vi "Configure Mask Test.vi"(0 "VISA resource name":refnum<visa-resource-name>, 1 "Enable Mask Test (Enable)":bool, 5 "Source (1: Channel 1)":i32(ring) items=["Channel 1", "Channel 2", "Channel 3", "Channel 4", "Function 1", "Function 2", "Function 3", "Function 4"], 7 "Trigger Source (1: Channel 1)":i32(ring) items=["Channel 1", "Channel 2", "Channel 3", "Channel 4"], 9 "Impedance (0: None)":i32(ring) items=["None", "IMP75", "IMP100", "IMP110", "IMP120"], 11 "error in (no error)":errorcluster, 12 "Run":T2 {"Time (1.0 min)" format="%#.1g"; "Run Mode (0: Forever)" items=["Forever", "Waveform", "Time"]}, 13 "Test Options":T3, 14 "Pulse Amplitude":T1) -> (4 "VISA resource name out":refnum<visa-resource-name>, 15 "error out":errorcluster)   [LabVIEW 2009, in "Agilent 8000 Series.lvlib"]
doc: "Configures the Mask test and the parameters required for a mask test. This VI has to be called before calling any other Mask related VIs."
uses:
  Agilent 8000 Series.lvlib
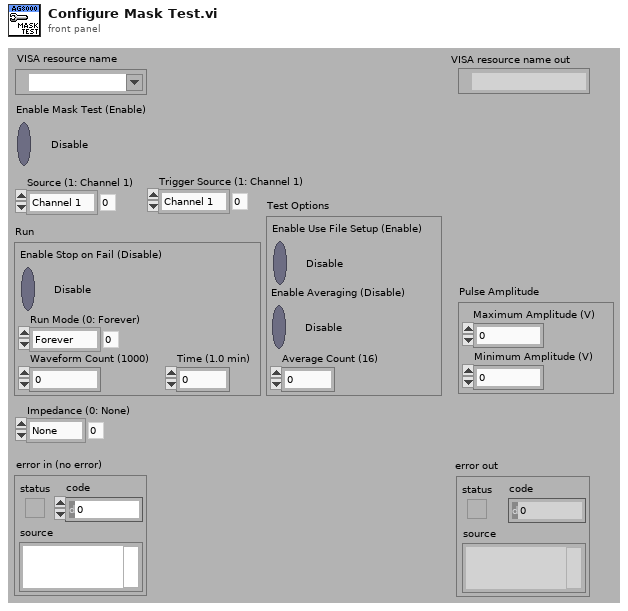
[diagram p1: front panel]
types:
  T1 = cluster{"Maximum Amplitude (V)":dbl, "Minimum Amplitude (V)":dbl}
  T2 = cluster{"Enable Stop on Fail (Disable)":bool, "Run Mode (0: Forever)":i32, "Waveform Count (1000)":u32, "Time (1.0 min)":dbl}
  T3 = cluster{"Enable Averaging (Disable)":bool, "Average Count (16)":u32, "Enable Use File Setup (Enable)":bool}
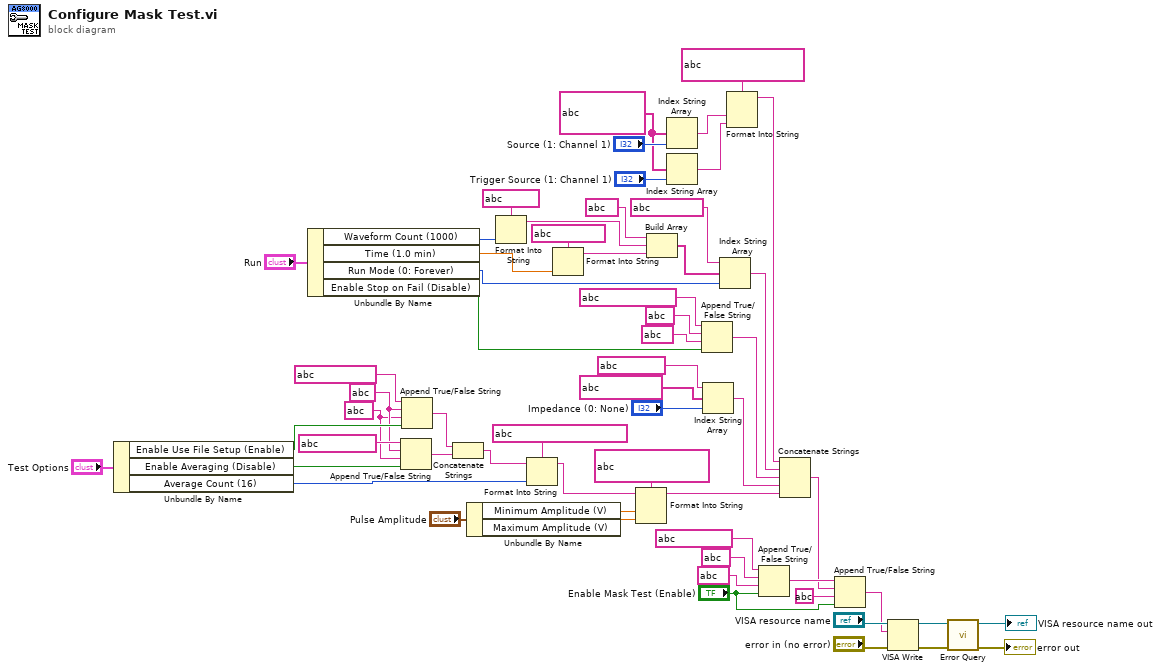
[diagram p0: block diagram]
diagram:
  w1 = string ? ("false string")
  w2 = string ? ("true string")
  w48 = string[] ?
  n1 = Unbundle By Name("Test Options") -> ("Enable Use File Setup (Enable)"=w6:bool, "Enable Averaging (Disable)"=w27:bool, "Average Count (16)"=w28:u32)
  n2 = Unbundle By Name("Run") -> ("Waveform Count (1000)"=w45:u32, "Time (1.0 min)"=w43:dbl, "Run Mode (0: Forever)"=w37:i32, "Enable Stop on Fail (Disable)"=w35:bool)
  n3 = Append True/False String(1:w27, 2:w1, 3:w2, 4:string ? ("string (\"\")")) -> (0:w3:string)
  n4 = Append True/False String(1:w6, 2:w1, 3:w2, 4:string ? ("string (\"\")")) -> (0:w5:string)
  n5 = Concatenate Strings(w5, w3) -> (w4:string)
  n6 = Unbundle By Name("Pulse Amplitude") -> ("Minimum Amplitude (V)"=w25:dbl, "Maximum Amplitude (V)"=w24:dbl)
  n7 = Format Into String(format string=string ?, w45) -> (resulting string=w40:string)  [unwired: 2 in, 1 out]
  n8 = Format Into String(format string=string ?, initial string=w4, w28) -> (resulting string=w20:string)  [unwired: 1 in, 1 out]
  n9 = Format Into String(format string=string ?, w43) -> (resulting string=w42:string)  [unwired: 2 in, 1 out]
  n10 = Format Into String(format string=string ?, initial string=w20, w25, w24) -> (resulting string=w18:string)  [unwired: 1 in, 1 out]
  n11 = Build Array(string ?, w40, w42) -> (w38:string[])
  n12 = Index String Array(1:"Source (1: Channel 1)", 2:w48) -> (0:w51:string)  [unwired: 1 in]
  n13 = Index String Array(1:"Trigger Source (1: Channel 1)", 2:w48) -> (0:w47:string)  [unwired: 1 in]
  n14 = Append True/False String(1:w35, 2:string ? ("false string"), 3:string ? ("true string"), 4:string ? ("string (\"\")")) -> (0:w19:string)
  n15 = Index String Array(1:"Impedance (0: None)", 2:string[] ? ("string array"), 3:string ? ("string (\"\")")) -> (0:w14:string)
  n16 = Index String Array(1:w37, 2:w38, 3:string ? ("string (\"\")")) -> (0:w21:string)
  n17 = Format Into String(format string=string ?, w51, w47) -> (resulting string=w22:string)  [unwired: 2 in, 1 out]
  n18 = Append True/False String(1:"Enable Mask Test (Enable)", 2:string ? ("false string"), 3:string ? ("true string"), 4:string ? ("string (\"\")")) -> (0:w11:string)
  n19 = Concatenate Strings(w22, w21, w19, w14, w18) -> (w10:string)
  n20 = Append True/False String(1:"Enable Mask Test (Enable)", 2:string ?, 3:w10, 4:w11) -> (0:w9:string)
  n21 = VISA Write(VISA resource name="VISA resource name", write buffer=w9, error in (no error)="error in (no error)") -> (VISA resource name out=w58:refnum<visa-resource-name>, error out=w57:errorcluster)  [unwired: 1 out]
  n22 = call "Error Query.vi"("error in (no error)"=w57, "VISA resource name"=w58) -> ("error out"=→"error out":errorcluster, "VISA resource name out"=→"VISA resource name out":refnum<visa-resource-name>)  [unwired: 6 in, 2 out]
